vi "emi_Tabs hidden.vi"(0 "Tab Control":refnum<vi>, 7 "Tabs to Grey out":i32[](array[numeric]), 11 "error in":errorcluster) -> (4 "Tab Control out":refnum<vi>, 15 "error out":errorcluster)   [LabVIEW 2010]
doc: "Setting tab visibility based on an array of indexes.\n\nOn error: do nothing."
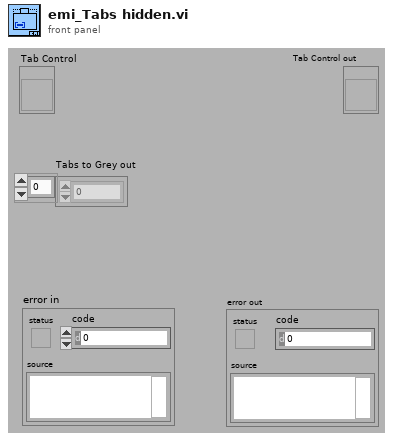
[diagram p1: front panel]
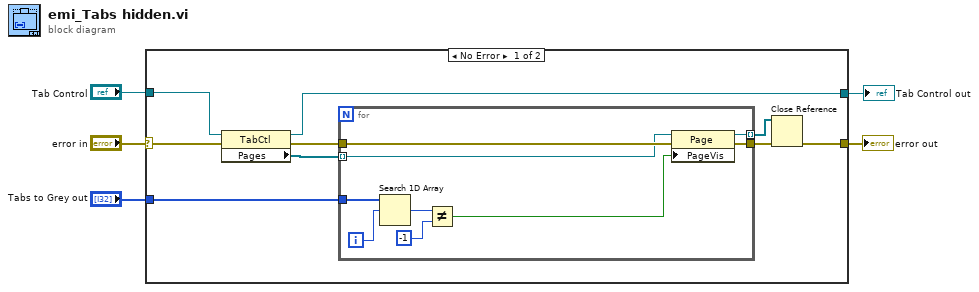
[diagram p0: block diagram]
diagram:
  n1 = case shown="No Error" "error in" {
    selector: "error in" -> [w7 w25]
    tunnel: "Tab Control" -> [w13 w24]
    tunnel: [w12 w24] -> w4
    tunnel: [w10 w25] -> w3
    tunnel: "Tabs to Grey out" -> [w6 _]
    frame No Error {
      n2 = property class="TabCtl"(reference=w13, error in=w7) -> (reference out=w12:refnum<vi>, error out=w14:errorcluster, "Pages"=w11:refnum<vi>[])
      n3 = for {
        tunnel: w14 -> [w23]
        tunnel: [w22] -> w9
        tunnel: w11 -> [w21] mode=indexing
        tunnel: [w20] -> w8 mode=indexing
        tunnel: w6 -> [w19]
        i -> [w18]
        n4 = Search 1D Array(1D array=w19, element=w18) -> (index of element=w17:i32)  [unwired: 1 in]
        n5 = Not Equal?(x=w17, y=-1) -> (x != y?=w15:bool)
        n6 = property class="Page"(reference=w21, error in=w23, "PageVis"=w15) -> (reference out=w20:refnum<vi>, error out=w22:errorcluster)
      }
      n7 = Close Reference(reference=w8, error in (no error)=w9) -> (error out=w10:errorcluster)
    }
    frame Error {
    }
  }
  "error out" <- w3
  "Tab Control out" <- w4
